vi "Display PCB coverage.vi"(0 "Inspection Data":T3, 5 "Dongle Fitted event Refnum in":T1, 11 "error in (no error)":errorcluster) -> (6 "Dongle fitted":bool, 15 "error out":errorcluster)   [LabVIEW 2013, in "Manipulate IPF.lvlib"]
uses:
  Manipulate IPF.lvlib
  type_def/but_exit.ctl
  3013/code/Modules/GUI/GUI_5/subPanels/edit/type_def/data.ctl
  3013/code/Modules/Configuration/type_def/Scan Params.ctl
  3013/code/Modules/Configuration/type_def/Profile Resolution.ctl
  3013/code/Modules/Preprocess Data/type_def/direction.ctl
  3013/code/Modules/Inspection/Data/Panel_class/type_def/Config File data.ctl
  3013/code/Modules/Inspection/type_def/Pos and Rot.ctl
  3013/code/Modules/Inspection/Data/PCB_class/type_def/PCB Params.ctl
  3013/code/Modules/Inspection/Data/Panel_class/type_def/BarCode Params.ctl
  3013/code/Modules/Barcode Reader/type_def/id.ctl
  3013/code/Modules/Inspection/Data/Panel_class/type_def/inspection data.ctl
  3013/code/Modules/Inspection/type_def/Range Limits.ctl
  Update TCF/type_def/Reload TCF_but.ctl
  type_def/Dongle fitted event refnum.ctl
  <vilib>/Utility/miscctls.llb/LVPointDoubleTypeDef.ctl
  <vilib>/Utility/cursorutil.llb/Set Cursor (Icon Pict).vi
  a3Di APG.lvlib
  3013/code/Modules/Inspection/Inspection.lvlib
  3013/code/Modules/Inspection/Data/PCB_class/PCB.lvclass
  3013/code/Modules/Barcode Reader/Barcode Reader.lvlib
  3013/code/Modules/Inspection/Data/Panel_class/Panel.lvclass
  3013/code/Modules/Configuration/Config.lvlib
  3013/code/Modules/Preprocess Data/PreProcess.lvlib
  3013/code/Modules/GUI/GUI_5/subPanels/edit/edit.lvlib
  Update TCF/TCF update.lvlib
panel:
  in  "Enable Labels":bool caption="Labels"
  out "XY Graph":cluster{dbl[], dbl[]}[](graph)
  in  "Enable Not Fited Components":bool caption="Not Fited Components"
  in  "Enable Not Tested Components":bool caption="Not Tested Components"
  in  "Save  to file":bool
  in  "Not Fitted Components":i32(listbox)
  in  "Not Tested Components":i32(listbox)
  in  "Reload":T2
  in  "Exit Button":T14
  # "Test Coverage\nComponents not tested (red), not fitted (green)"
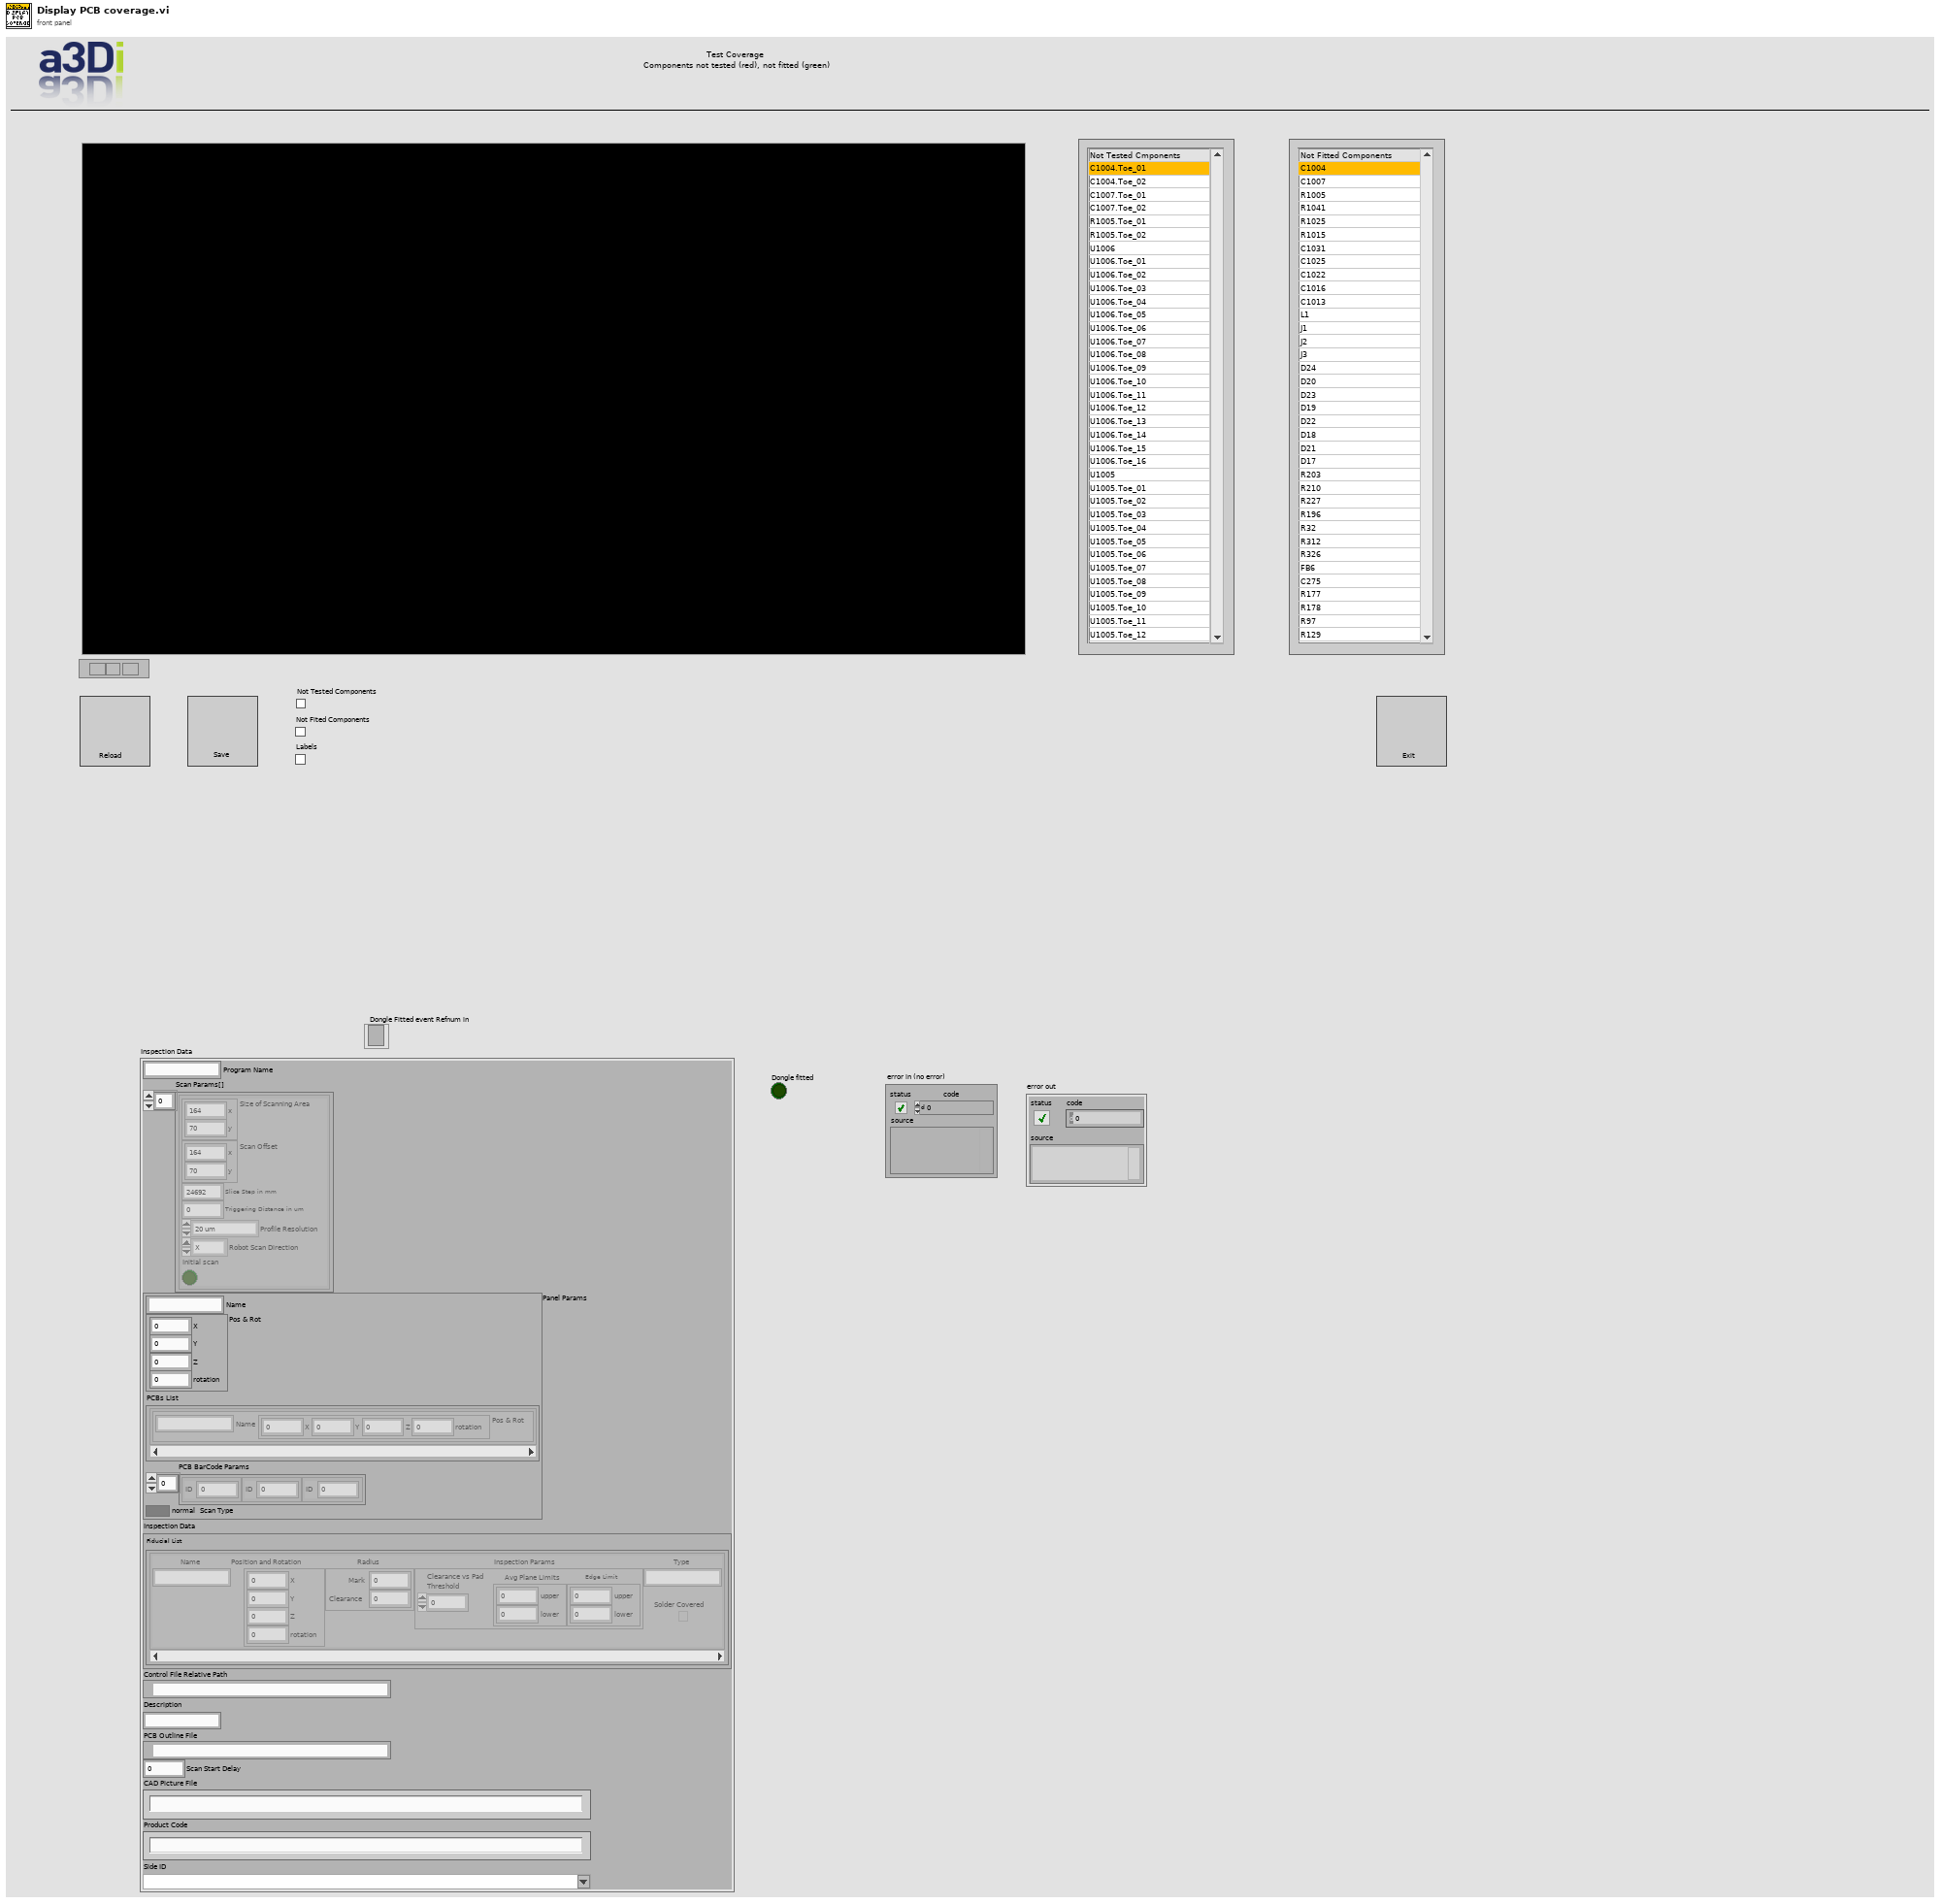
[diagram p1: front panel]
types:
  T1 = typedef "Dongle fitted event refnum.ctl" = refnum<event-registration>
  T2 = typedef "TCF update.lvlib/Reload TCF_but.ctl" = bool
  T3 = typedef "GUI.lvlib/subPanel.lvlib/edit.lvlib/data.ctl" = cluster{"Program Name":string, "Scan Params[]":T4[], "Panel Params":T7, "Inspection Data":T12, "Control File Relative Path":path, "Description":string, "PCB Outline File":path, "Scan Start Delay":dbl, "CAD Picture File":string, "Product Code":string, "Side ID":string}
  T4 = typedef "Config.lvlib/Scan Params.ctl" = cluster{"Size of Scanning Area":cluster{"x":dbl, "y":dbl}, "Scan Offset":cluster{"x":dbl, "y":dbl}, "Slice Step in mm":dbl, "Triggering Distance in mm":dbl, "Triggering Distance in um":dbl, "Profile Resolution":T5, "Version":string, "Robot Scan Direction":T6, "Initial scan":bool}
  T5 = typedef "Config.lvlib/Profile Resolution.ctl" = enum8{"20 um", "40 um"}
  T6 = typedef "PreProcess.lvlib/direction.ctl" = enum8{"X", "Y"}
  T7 = typedef "Inspection.lvlib/Panel.lvclass/Config File data.ctl" = cluster{"Name":string, "Pos & Rot":T8, "PCBs List":cluster{"PCB Params":T9}[], "PCB BarCode Params":T10[], "Scan Type":bool}
  T8 = typedef "Inspection.lvlib/Pos and Rot.ctl" = cluster{"X":dbl, "Y":dbl, "Z":dbl, "rotation":dbl}
  T9 = typedef "Inspection.lvlib/PCB.lvclass/PCB Params.ctl" = cluster{"Name":string, "Pos & Rot":T8}
  T10 = typedef "Inspection.lvlib/Panel.lvclass/BarCode Params.ctl" = cluster{"ID":T11}
  T11 = typedef "Barcode Reader.lvlib/id.ctl" = u8
  T12 = typedef "Inspection.lvlib/Panel.lvclass/inspection data.ctl" = cluster{"Fiducial List":cluster{"Name":string, "Position and Rotation":T8, "Radius":cluster{"Mark":dbl, "Clearance":dbl}, "Inspection Params":cluster{"Clearance vs Pad\nThreshold":dbl, "Avg Plane Limits":T13, "Edge Limit":T13}, "Type":string, "Solder Covered":bool}[]}
  T13 = typedef "Inspection.lvlib/Range Limits.ctl" = cluster{"upper":sgl, "lower":sgl}
  T14 = typedef "a3Di APG.lvlib/but_exit.ctl" = bool
  T15 = enum16{"Initialisation", "Wait for user input", "Scale changed", "Exit"}
  T16 = cluster{"Enable Not Tested Components":bool, "Enable Not Fited Components":bool, "Enable Labels":bool}
  T17 = enum32{"Invalid", "Standard", "Closed", "Hidden", "Minimized", "Maximized"}
  T18 = typedef "LVPointDoubleTypeDef.ctl" = cluster{"X":dbl, "Y":dbl}
  T19 = cluster{"XScale.Max":dbl, "XScale.Min":dbl, "YScale.Max":dbl, "YScale.Min":dbl}
  T20 = cluster{"Not fitted components":string[], "Not tested components":string[], "Not Fitted position[x][y] ":dbl[][], "Not Tested position[x][y]":dbl[][], "CAD Layers":cluster{"1st Filtered Array out":sgl[], "2nd Filtered Array out":sgl[]}[], "Xyz File Exist? ":bool, "Options":cluster{"Enable Not Tested Components":bool, "Enable Not Fited Components":bool, "Enable Labels":bool}, "Origin XY Scale Ranges":cluster{"XScale.Max":dbl, "XScale.Min":dbl, "YScale.Max":dbl, "YScale.Min":dbl}}
  T21 = typedef "LVPoint32TypeDef.ctl" = cluster{"Horizontal":i32, "Vertical":i32}
  T22 = cluster{"XScale.Offset":dbl, "YScale.Offset":dbl}
  T23 = cluster{"XScale.Multiplier":dbl, "YScale.Multiplier":dbl}
  T24 = typedef "LVAnnotationListTypeDef.ctl" = cluster{"Name":string, "Color":u32, "Style":u8, "Point Style":u8, "Name Visible":bool, "Allow Drag":bool, "Annotation Mode":u32, "Plot":i32, "Index":i32, "Position":cluster{"X":dbl, "Y":dbl}, "X Scale":u32, "Y Scale":u32, "Show Arrow":bool, "Lock Name":bool, "Plot Area":i32, "Label Offset":cluster{"X":dbl, "Y":dbl}}[]
  T25 = cluster{"Name":string, "Color":u32, "Style":u8, "Point Style":u8, "Name Visible":bool, "Allow Drag":bool, "Annotation Mode":u32, "Plot":i32, "Index":i32, "Position":cluster{"X":dbl, "Y":dbl}, "X Scale":u32, "Y Scale":u32, "Show Arrow":bool, "Lock Name":bool, "Plot Area":i32, "Label Offset":cluster{"X":dbl, "Y":dbl}}
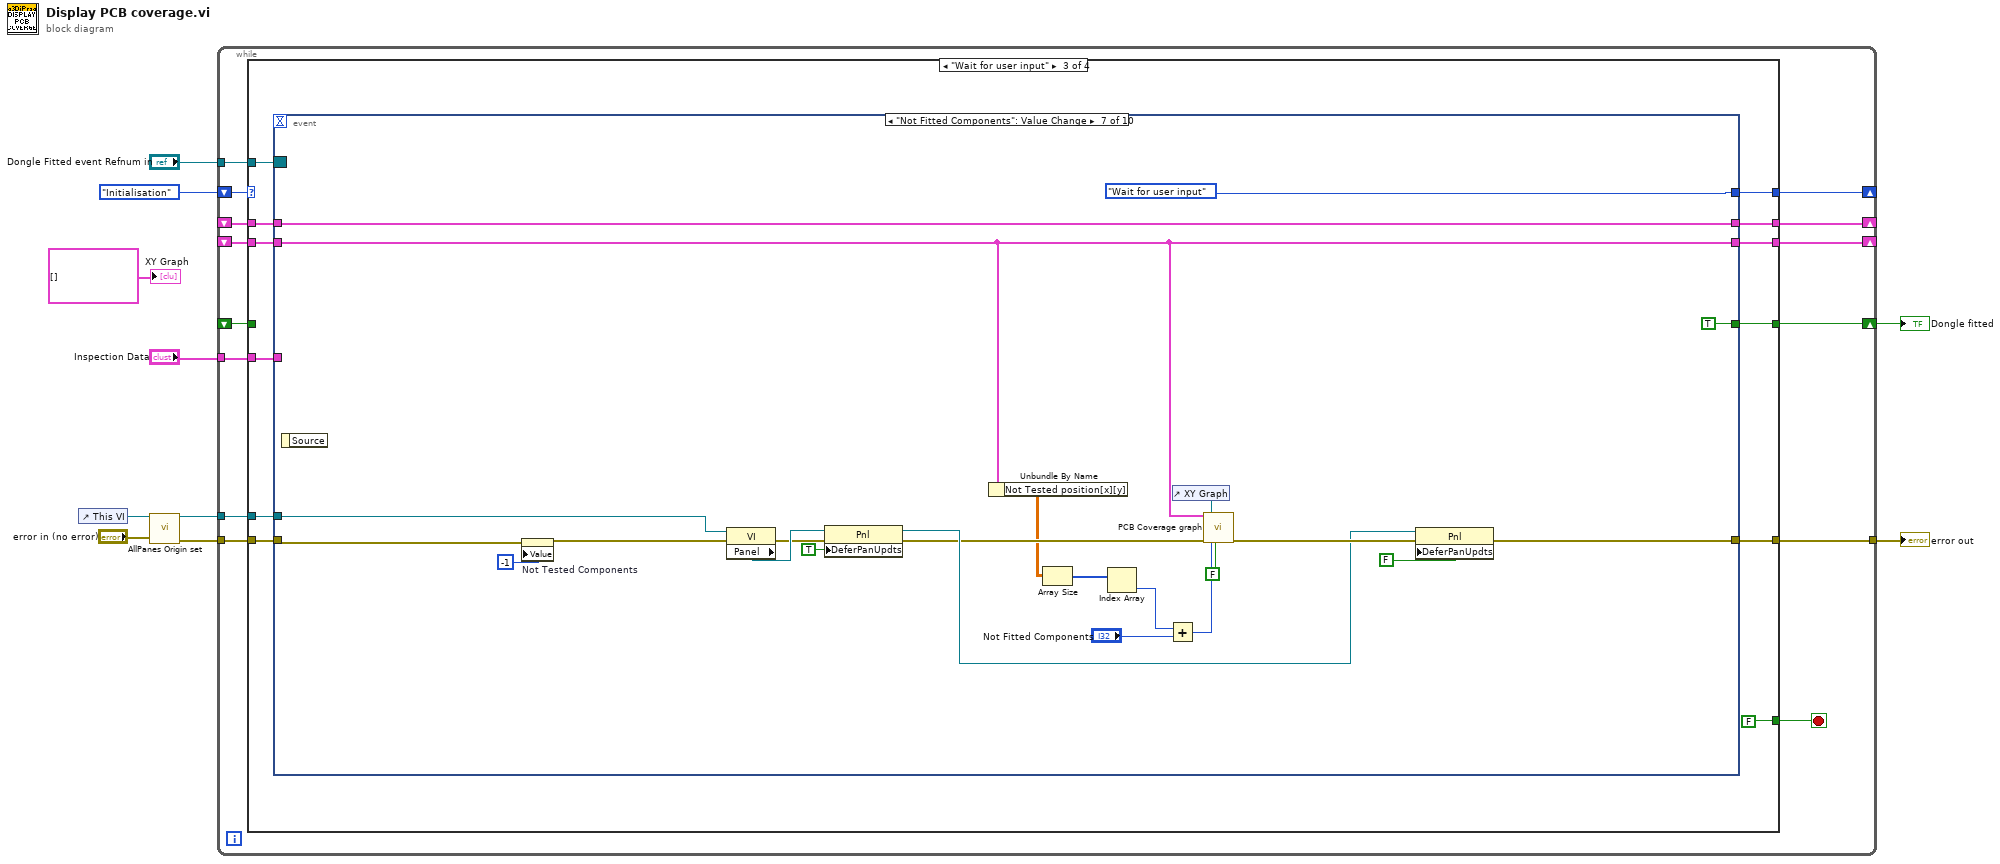
[diagram p0: block diagram]
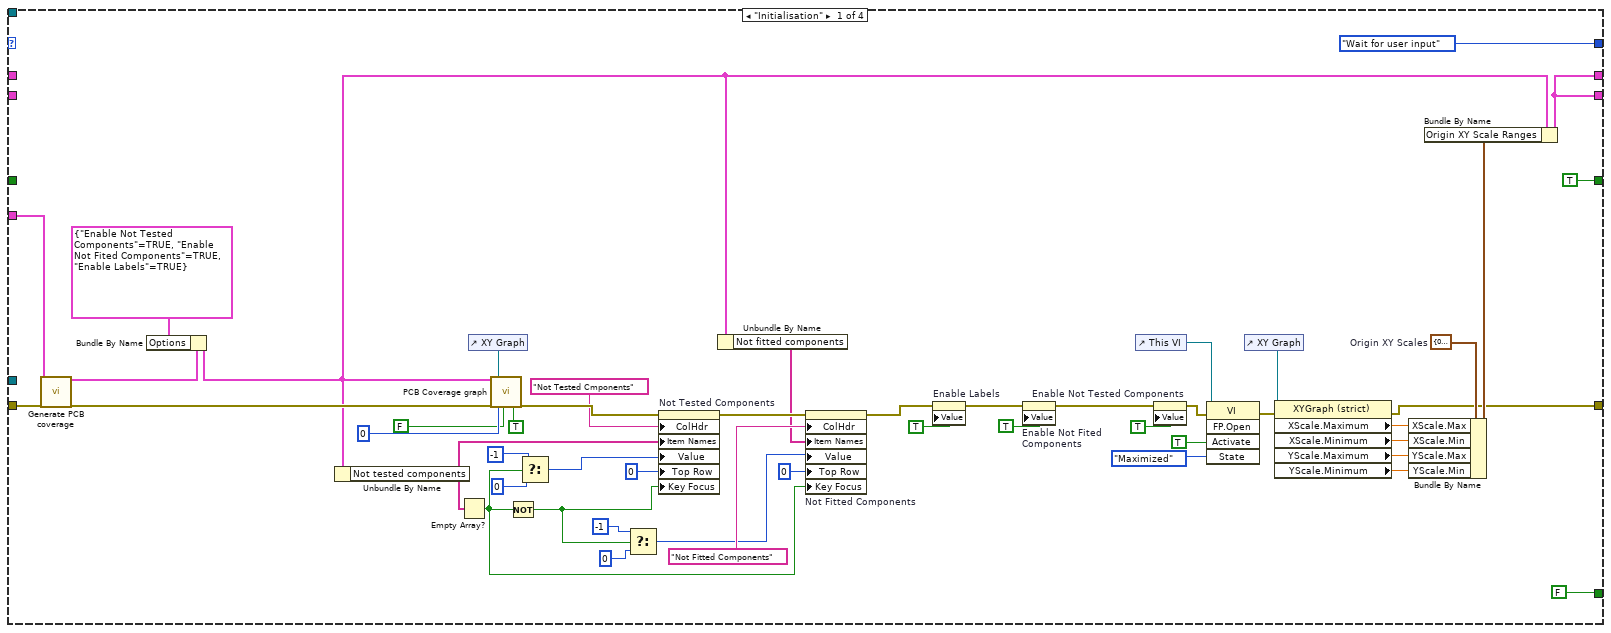
[diagram p2: hidden frame]
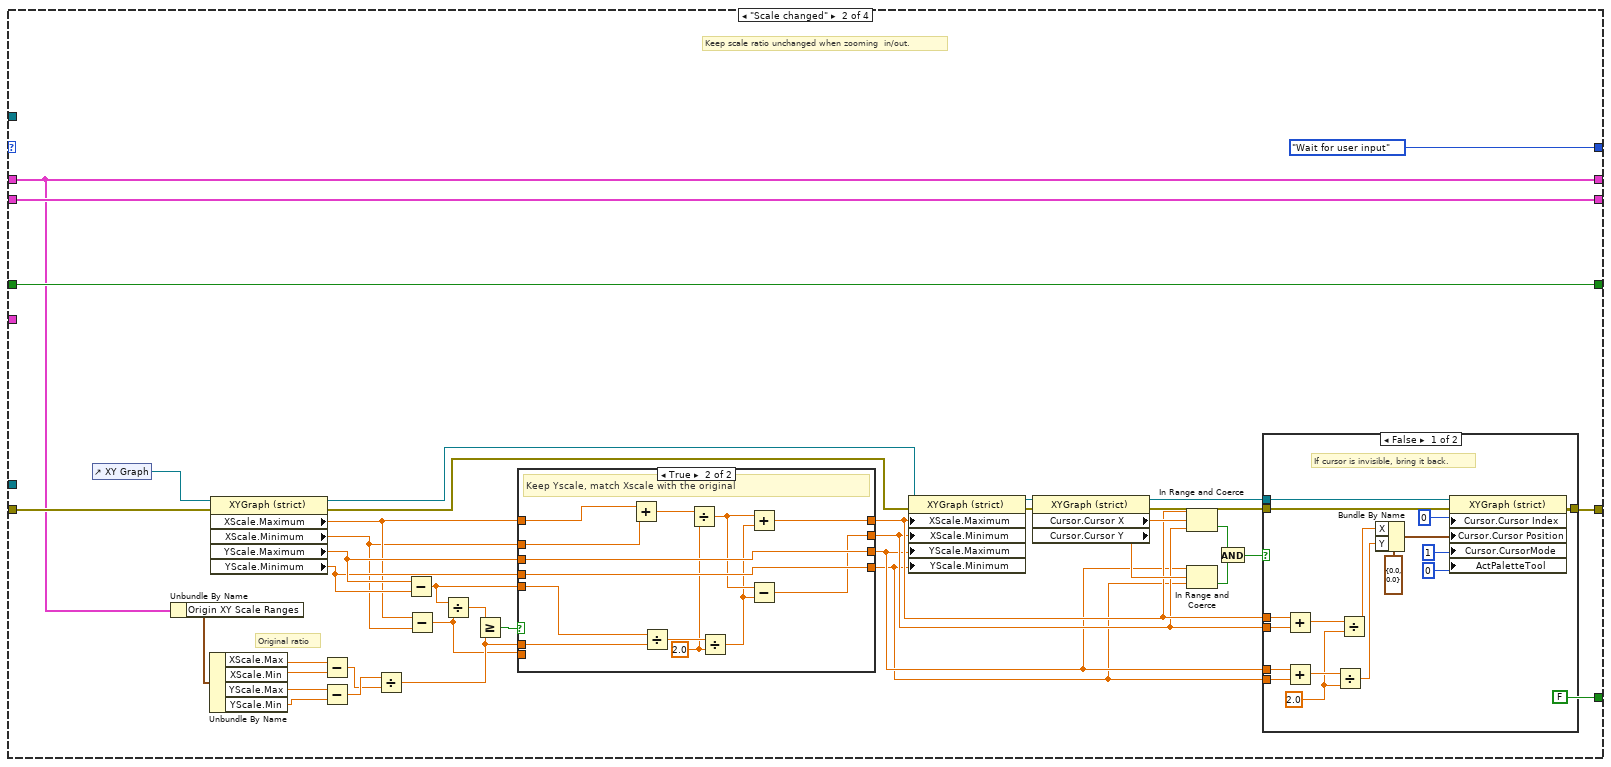
[diagram p3: hidden frame]
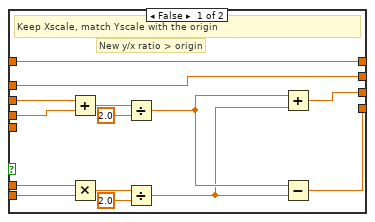
[diagram p5: hidden frame]
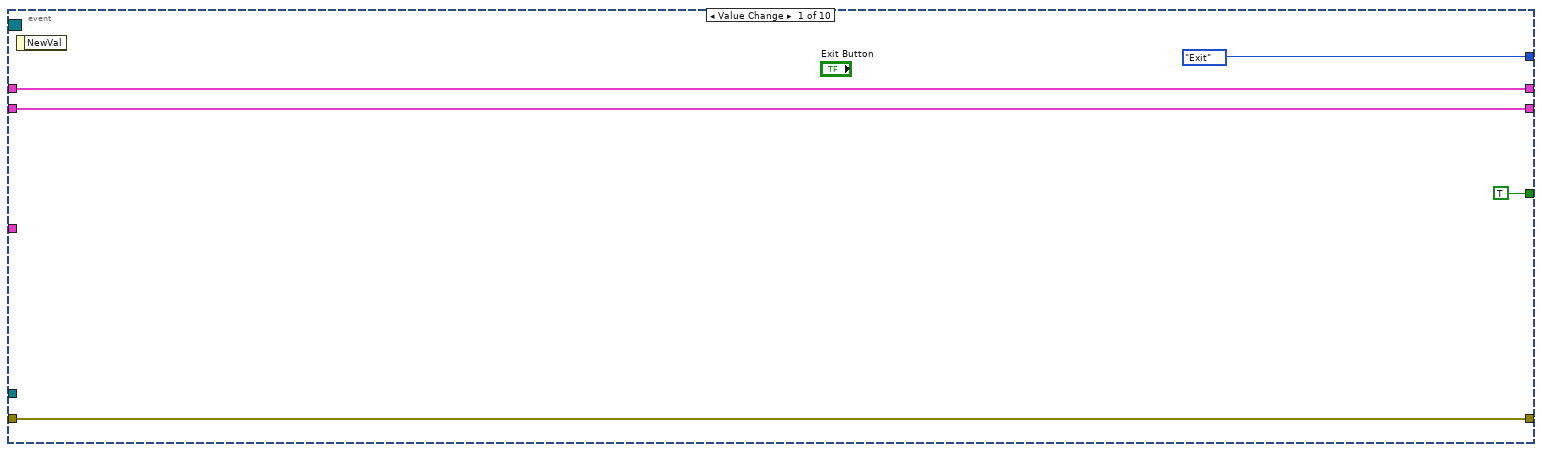
[diagram p6: hidden frame]
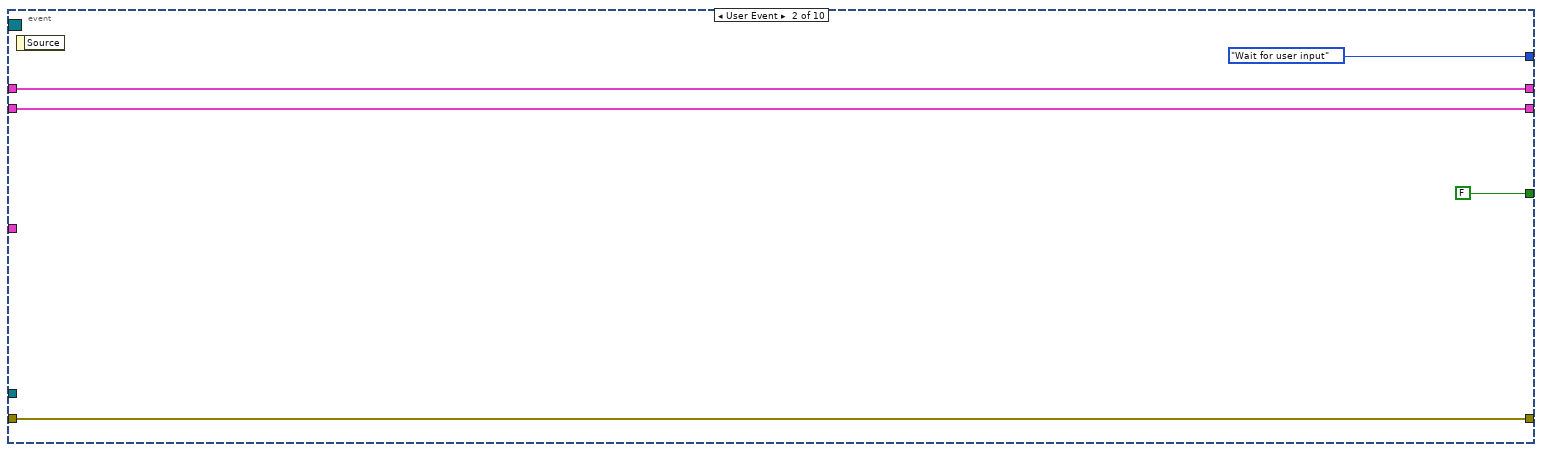
[diagram p7: hidden frame]
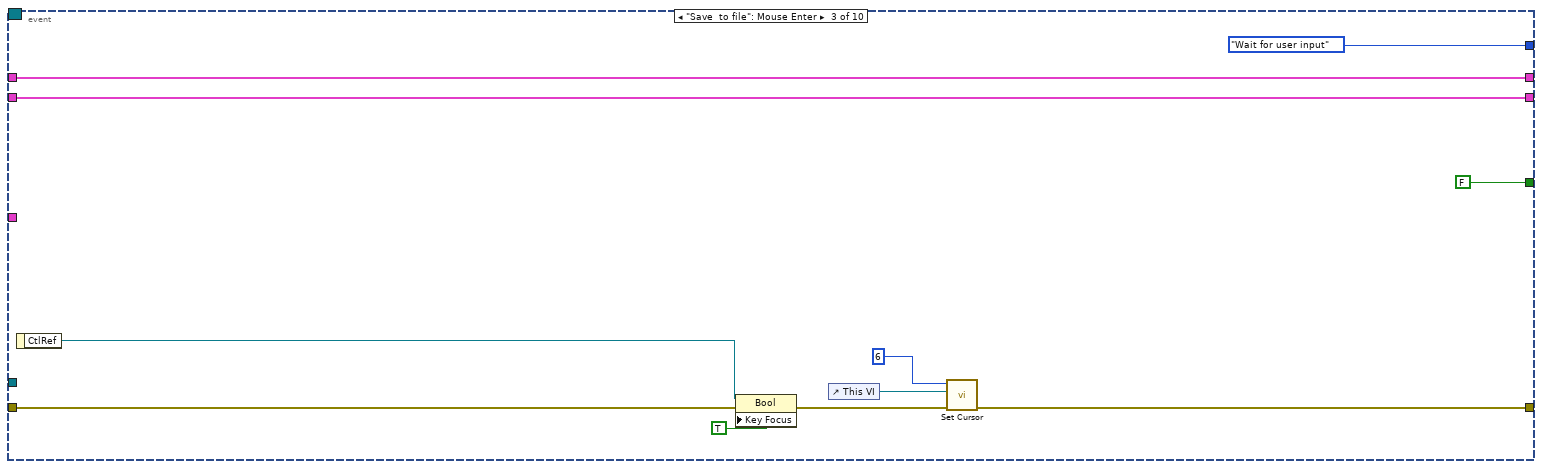
[diagram p8: hidden frame]
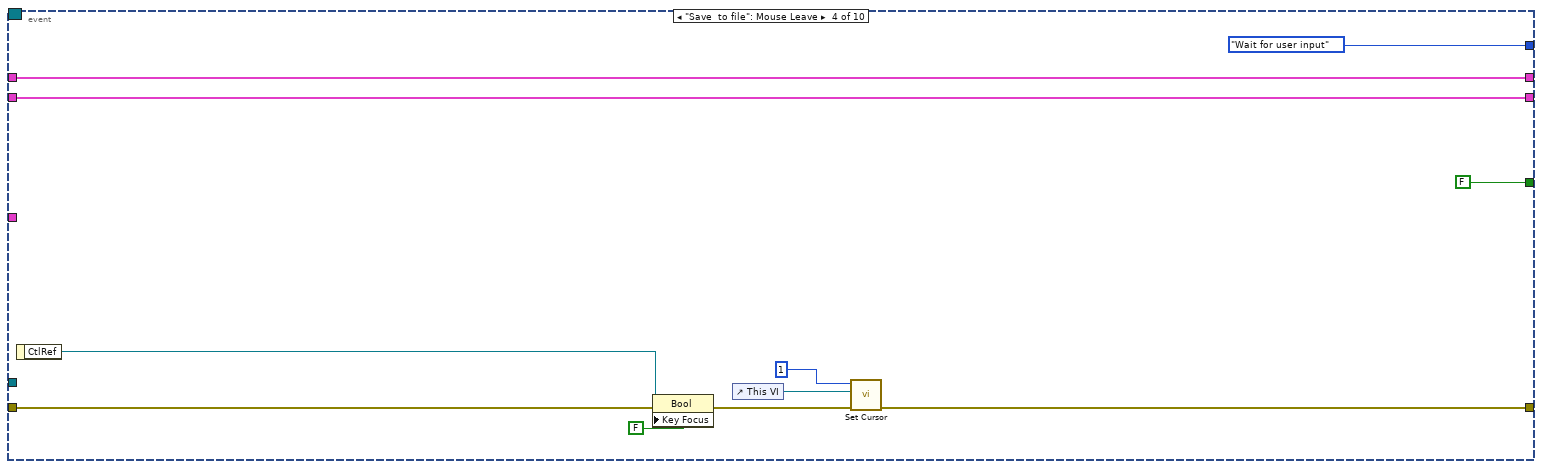
[diagram p9: hidden frame]
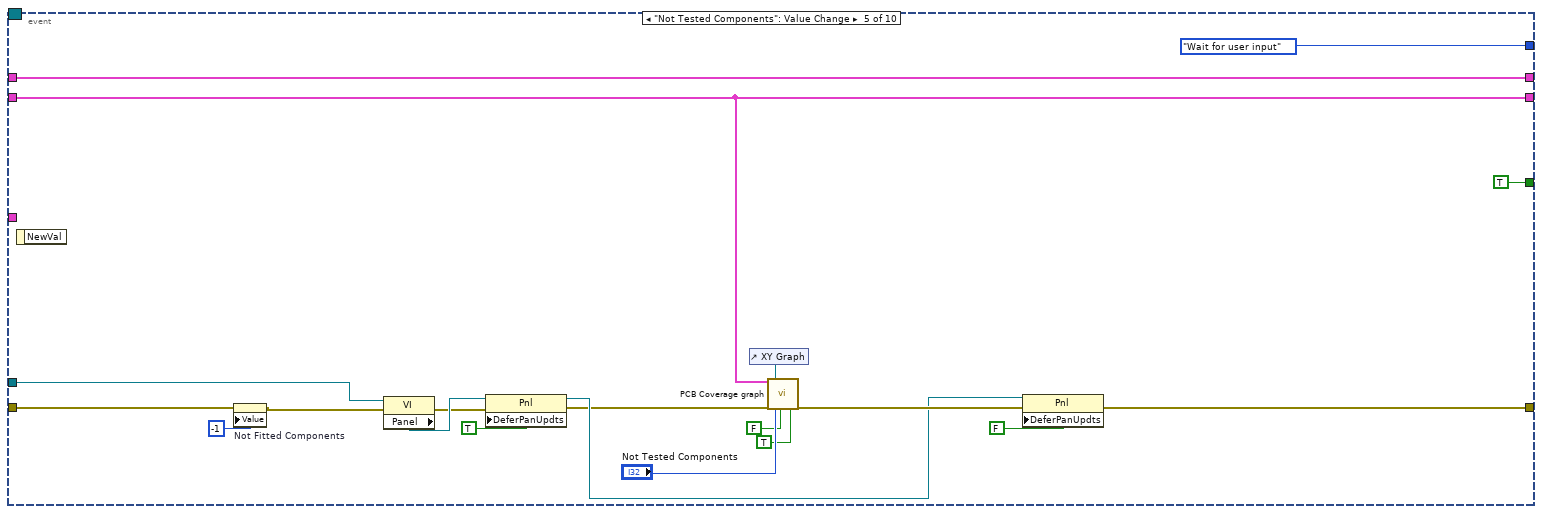
[diagram p10: hidden frame]
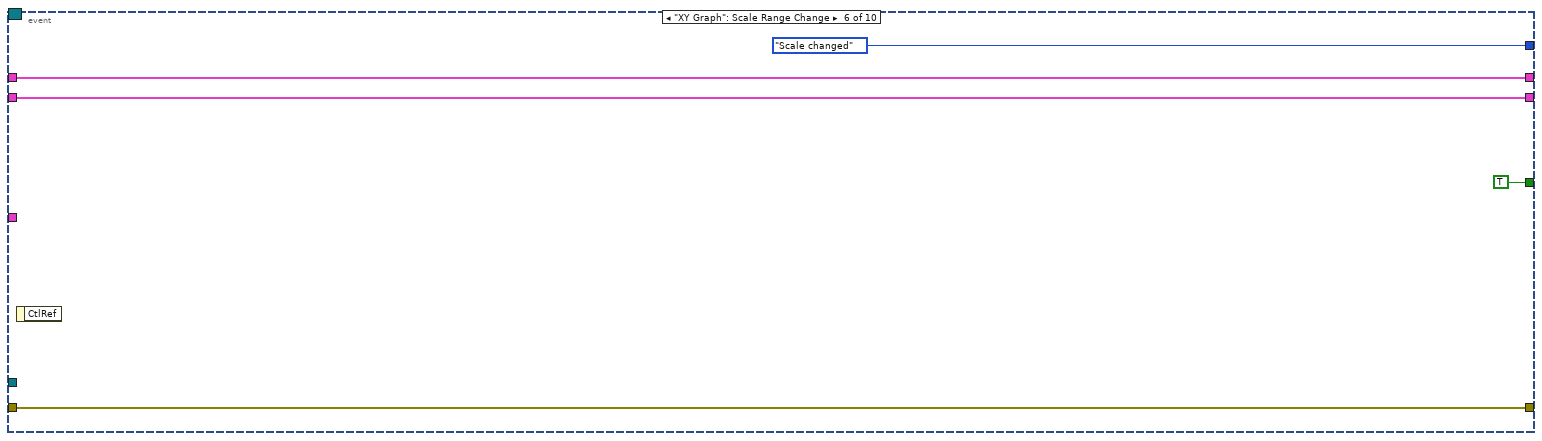
[diagram p11: hidden frame]
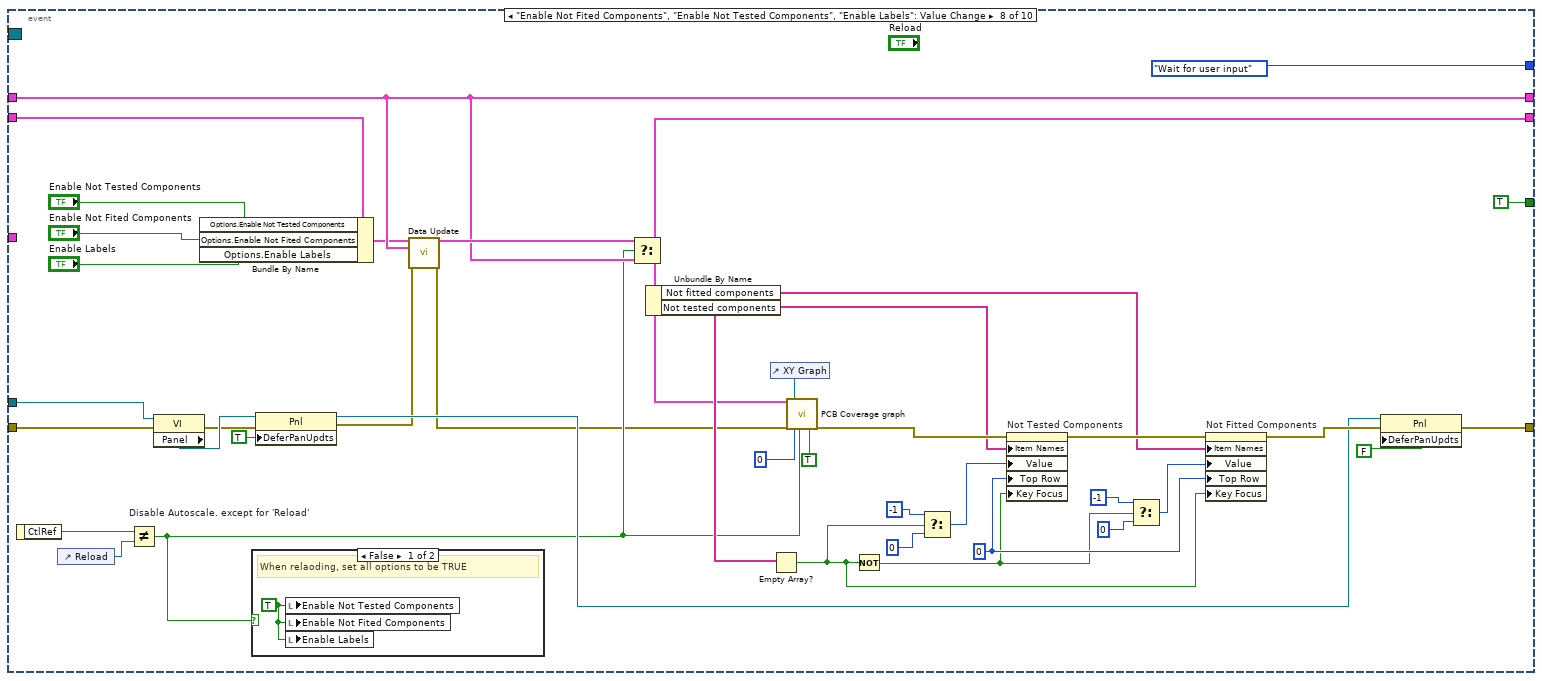
[diagram p12: hidden frame]
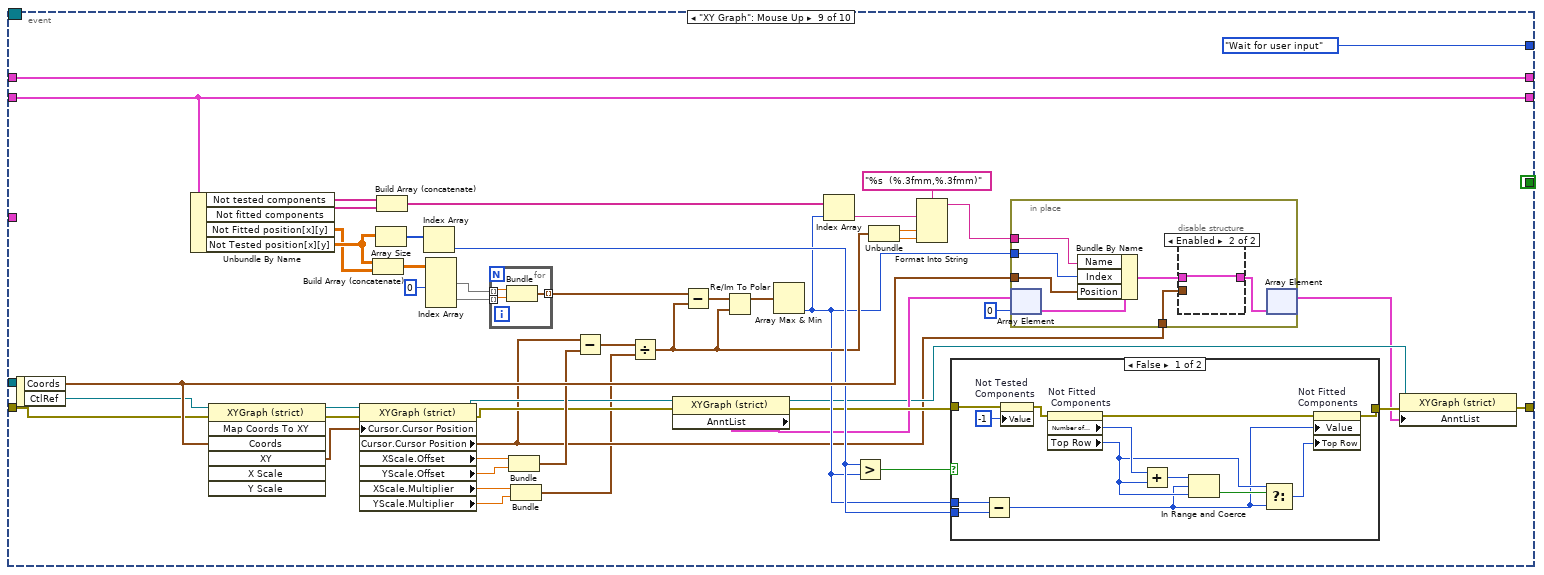
[diagram p14: hidden frame]
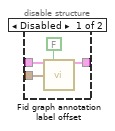
[diagram p15: hidden frame]
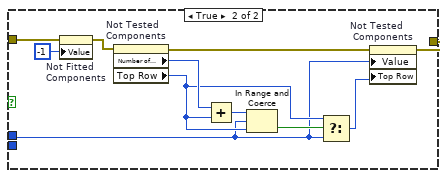
[diagram p16: hidden frame]
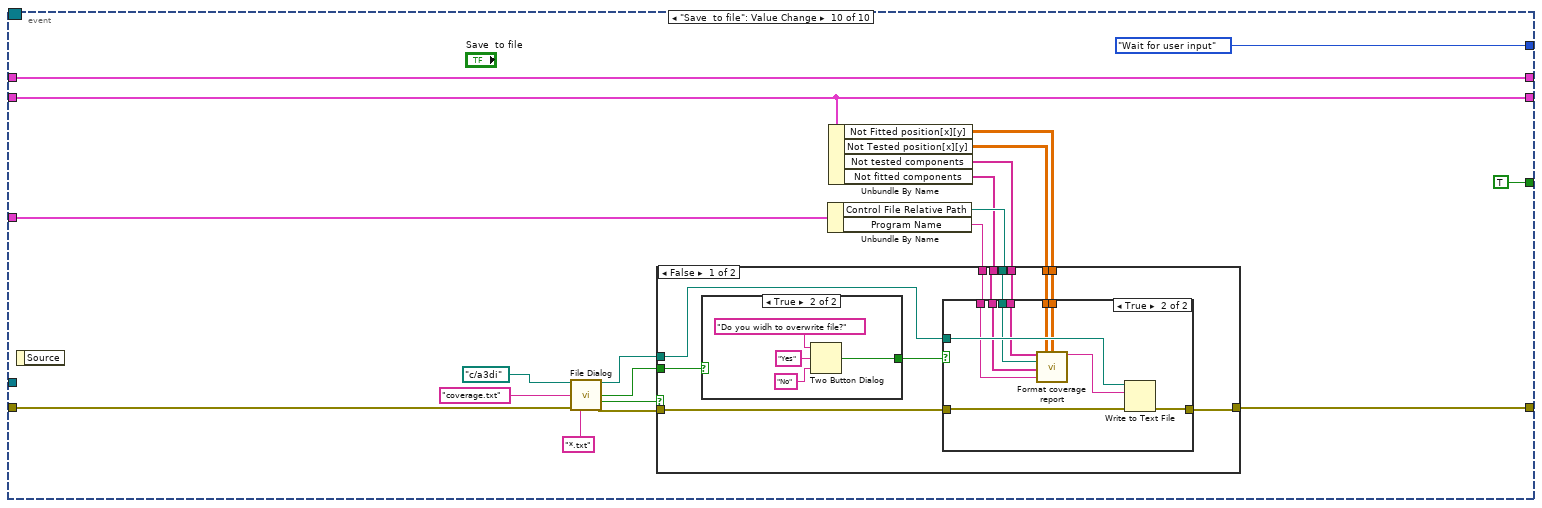
[diagram p17: hidden frame]
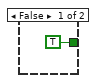
[diagram p19: hidden frame]
diagram:
  n1 = control-ref of="This VI"() -> (w10:refnum<vi>)
  n2 = call "AllPanes Origin set.vi"("VI ref in"=w10, "error in"="error in (no error)") -> ("VI ref out"=w7:refnum<vi>, "error out"=w8:errorcluster)  [unwired: 12 in]
  n3 = while {
    tunnel: w8 -> [w22]
    shift-right: [w23] -> _
    shift-left: T15."Initialisation" -> [w24]
    tunnel: [w19] -> w1
    tunnel: w7 -> [w21]
    tunnel: "Inspection Data" -> [w20]
    tunnel: "Dongle Fitted event Refnum in" -> [w18]
    shift-right: [w17] -> w4
    shift-left: _ -> [w16]
    shift-right: [w15] -> _
    shift-left: _ -> [w14]
    shift-right: [w12] -> _
    shift-left: _ -> [w13]
    stop <- w11 stop-if-true
    n4 = case shown="\"Wait for user input\"" w24 {
      tunnel: [FALSE FALSE FALSE TRUE] -> w11
      tunnel: [T15."Wait for user input" T15."Wait for user input" w169 T15."Exit"] -> w23
      tunnel: w22 -> [w34 w109 w167 w433]
      tunnel: [w25 w87 w158 w427] -> w19
      tunnel: w21 -> [_ _ w163 w432]
      tunnel: w20 -> [w69 _ w168 _]
      tunnel: w18 -> [_ _ w165 _]
      tunnel: [TRUE w111 w164 w431] -> w17
      tunnel: w16 -> [_ w111 _ w431]
      tunnel: [w27 w107 w161 w429] -> w15
      tunnel: w14 -> [_ w107 w162 w429]
      tunnel: w13 -> [_ w108 w159 w428]
      tunnel: [w27 w108 w160 w428] -> w12
      frame "Initialisation" {
        w41 = T19 {"XScale.Max"=0.0, "XScale.Min"=0.0, "YScale.Max"=0.0, "YScale.Min"=0.0}  # Origin XY Scales
        n5 = call "Generate PCB coverage.vi"("Inspection Data"=w69, "error in (no error)"=w34) -> ("DataOut"=w31:T20, "error out"=w68:errorcluster)  [unwired: 16 in]
        n6 = Bundle By Name(cluster=w31, "Options"=T16 {"Enable Not Tested Components"=TRUE, "Enable Not Fited Components"=TRUE, "Enable Labels"=TRUE}) -> (w29:T20)
        n7 = Unbundle By Name(w29) -> ("Not tested components"=w28:string[])
        n8 = Empty Array?(array=w28) -> (empty?=w54:bool)
        n9 = control-ref of="XY Graph"() -> (w47:refnum<vi>)
        n10 = call "PCB Coverage graph.vi"("UpdatedData"=w29, "error in (no error)"=w68, "XY Graph"=w47, "index"=0, "Disable Autoscale"=FALSE ("Disable Zoom Back?"), "Initialise graph"=TRUE) -> ("error out"=w67:errorcluster)  [unwired: 13 in]
        n11 = Not(x=w54) -> (.not. x?=w57:bool)
        n12 = Select(t=-1 ("Not Tested Components"), s=w54, f=0 ("Not Tested Components")) -> (s? t:f=w59:i32)
        n13 = Select(t=-1 ("Not Tested Components"), s=w57, f=0 ("Not Tested Components")) -> (s? t:f=w55:i32)
        n14 = property on="Not Tested Components" class="LstBox (strict)"(error in=w67, "ColHdr"="Not Tested Cmponents" ("Column Header String"), "Item Names"=w28, "Value"=w59, "Top Row"=0 ("Not Tested Components"), "Key Focus"=w57) -> (error out=w66:errorcluster)  [unwired: 1 in, 1 out]
        n15 = Unbundle By Name(w29) -> ("Not fitted components"=w30:string[])
        n16 = property on="Not Fitted Components" class="LstBox (strict)"(error in=w66, "ColHdr"="Not Fitted Components" ("Column Header String"), "Item Names"=w30, "Value"=w55, "Top Row"=0 ("Not Fitted Components"), "Key Focus"=w54) -> (error out=w46:errorcluster)  [unwired: 1 in, 1 out]
        n17 = property on="Enable Labels" class="Bool (strict)"(error in=w46, "Value"=TRUE ("Enable Labels")) -> (error out=w45:errorcluster)  [unwired: 1 in, 1 out]
        n18 = property on="Enable Not Fited Components" class="Bool (strict)"(error in=w45, "Value"=TRUE ("Not Fited Components")) -> (error out=w49:errorcluster)  [unwired: 1 in, 1 out]
        n19 = control-ref of="This VI"() -> (w70:refnum<vi>)
        n20 = property on="Enable Not Tested Components" class="Bool (strict)"(error in=w49, "Value"=TRUE ("Not Fited Components")) -> (error out=w48:errorcluster)  [unwired: 1 in, 1 out]
        n21 = invoke class="VI" method="FP.Open"(reference=w70, error in=w48, "Activate"=TRUE ("Activate?"), "State"=T17."Maximized") -> (error out=w35:errorcluster)  [unwired: 1 in, 4 out]
        n22 = control-ref of="XY Graph"() -> (w42:refnum<vi>)
        n23 = property class="XYGraph (strict)"(reference=w42, error in=w35) -> (error out=w25:errorcluster, "XScale.Maximum"=w40:dbl, "XScale.Minimum"=w39:dbl, "YScale.Maximum"=w38:dbl, "YScale.Minimum"=w37:dbl)  [unwired: 1 out]
        n24 = Bundle By Name(cluster=w41, "XScale.Max"=w40, "XScale.Min"=w39, "YScale.Max"=w38, "YScale.Min"=w37) -> (w26:T19)
        n25 = Bundle By Name(cluster=w29, "Origin XY Scale Ranges"=w26) -> (w27:T20)
      }
      frame "Scale changed" {
        # "Original ratio"
        # "Keep scale ratio unchanged when zooming  in/out."
        n26 = control-ref of="XY Graph"() -> (w106:refnum<vi>)
        n27 = Unbundle By Name(w107) -> ("Origin XY Scale Ranges"=w88:T19)
        n28 = Unbundle By Name(w88) -> ("XScale.Max"=w104:dbl, "XScale.Min"=w103:dbl, "YScale.Max"=w102:dbl, "YScale.Min"=w101:dbl)
        n29 = property class="XYGraph (strict)"(reference=w106, error in=w109) -> (reference out=w105:refnum<vi>, error out=w89:errorcluster, "XScale.Maximum"=w94:dbl, "XScale.Minimum"=w93:dbl, "YScale.Maximum"=w96:dbl, "YScale.Minimum"=w95:dbl)
        n30 = Subtract(x=w104, y=w103) -> (x-y=w99:dbl)
        n31 = Subtract(x=w102, y=w101) -> (x-y=w100:dbl)
        n32 = Divide(x=w100, y=w99) -> (x/y=w92:dbl)
        n33 = Subtract(x=w96, y=w95) -> (x-y=w91:dbl)
        n34 = Subtract(x=w94, y=w93) -> (x-y=w90:dbl)
        n35 = Divide(x=w91, y=w90) -> (x/y=w98:dbl)
        n36 = Greater Or Equal?(x=w98, y=w92) -> (x >= y?=w97:bool)
        n37 = case shown="True" w97 {
          tunnel: w96 -> [w137 w157]
          tunnel: [w142 w157] -> w78
          tunnel: [w131 w156] -> w77
          tunnel: w95 -> [w136 w156]
          tunnel: w94 -> [w144 w152]
          tunnel: [w144 w149] -> w80
          tunnel: w93 -> [w143 w151]
          tunnel: [w143 w146] -> w79
          tunnel: w92 -> [w140 w154]
          tunnel: w91 -> [_ w155]
          tunnel: w90 -> [w141 _]
          frame False {
            # "New y/x ratio > origin"
            # "Keep Xscale, match Yscale with the origin"
            n38 = Add(x=w137, y=w136) -> (x+y=w134:dbl)
            n39 = Multiply(x=w140, y=w141) -> (x*y=w139:dbl)
            n40 = Divide(x=w134, y=2.0) -> (x/y=w133:dbl)
            n41 = Divide(x=w139, y=2.0) -> (x/y=w132:dbl)
            n42 = Add(x=w133, y=w132) -> (x+y=w142:dbl)
            n43 = Subtract(x=w133, y=w132) -> (x-y=w131:dbl)
          }
          frame True {
            w145 = 2.0 ("y")
            # "Keep Yscale, match Xscale with the original"
            n44 = Add(x=w152, y=w151) -> (x+y=w150:dbl)
            n45 = Divide(x=w155, y=w154) -> (x/y=w153:dbl)
            n46 = Divide(x=w150, y=w145) -> (x/y=w148:dbl)
            n47 = Divide(x=w153, y=w145) -> (x/y=w147:dbl)
            n48 = Add(x=w148, y=w147) -> (x+y=w149:dbl)
            n49 = Subtract(x=w148, y=w147) -> (x-y=w146:dbl)
          }
        }
        n50 = property class="XYGraph (strict)"(reference=w105, error in=w89, "XScale.Maximum"=w80, "XScale.Minimum"=w79, "YScale.Maximum"=w78, "YScale.Minimum"=w77) -> (reference out=w86:refnum<vi>, error out=w84:errorcluster)
        n51 = property class="XYGraph (strict)"(reference=w86, error in=w84) -> (reference out=w85:refnum<vi>, error out=w83:errorcluster, "Cursor.Cursor X"=w82:dbl, "Cursor.Cursor Y"=w81:dbl)
        n52 = In Range and Coerce(upper limit=w80, x=w82, lower limit=w79) -> (In Range?=w76:bool)  [unwired: 1 out]
        n53 = In Range and Coerce(upper limit=w78, x=w81, lower limit=w77) -> (In Range?=w75:bool)  [unwired: 1 out]
        n54 = And(x=w76, y=w75) -> (x .and. y?=w74:bool)
        n55 = case shown="False" w74 {
          tunnel: w80 -> [w124 _]
          tunnel: w79 -> [w123 _]
          tunnel: w78 -> [w119 _]
          tunnel: w77 -> [w118 _]
          tunnel: [w116 w130] -> w87
          tunnel: w85 -> [w114 _]
          tunnel: w83 -> [w113 w130]
          frame False {
            w115 = 2.0 ("y")
            # "If cursor is invisible, bring it back."
            n56 = Add(x=w124, y=w123) -> (x+y=w122:dbl)
            n57 = Add(x=w119, y=w118) -> (x+y=w120:dbl)
            n58 = Divide(x=w120, y=w115) -> (x/y=w117:dbl)
            n59 = Divide(x=w122, y=w115) -> (x/y=w121:dbl)
            n60 = Bundle By Name(cluster=T18 {"X"=0.0, "Y"=0.0} ("Cursor.Cursor Position"), "X"=w121, "Y"=w117) -> (w126:T18)
            n61 = property class="XYGraph (strict)"(reference=w114, error in=w113, "Cursor.Cursor Index"=0, "Cursor.Cursor Position"=w126, "Cursor.CursorMode"=u32 1 ("Cursor.Cursor Mode"), "ActPaletteTool"=0 ("Palette:Active Tool")) -> (error out=w116:errorcluster)  [unwired: 1 out]
          }
          frame True {
          }
        }
      }
      frame "Wait for user input" {
        n62 = event shown="[6] \"Not Fitted Components\": Value Change" {
          selector: w165 -> [_ _ _ _ _ _ _ _ _ _]
          dyn-events: _ -> [_ _ _ _ _ _ _ _ _ _]
          timeout: _ -> [_ _ _ _ _ _ _ _ _ _]
          tunnel: [T15."Exit" T15."Wait for user input" T15."Wait for user input" T15."Wait for user input" T15."Wait for user input" T15."Scale changed" T15."Wait for user input" T15."Wait for user input" T15."Wait for user input" T15."Wait for user input"] -> w169
          tunnel: w168 -> [_ _ _ _ _ _ _ _ _ w389]
          tunnel: w167 -> [w174 w179 w181 w192 w210 w222 w235 w252 w291 w398]
          tunnel: [w174 w179 w185 w196 w214 w222 w239 w284 w292 w393] -> w158
          tunnel: w163 -> [_ _ _ _ w216 _ w241 w289 _ _]
          tunnel: [TRUE FALSE FALSE FALSE TRUE TRUE TRUE TRUE TRUE TRUE] -> w164
          tunnel: w162 -> [w171 w176 w188 w199 w202 w224 w229 w260 w336 w384]
          tunnel: [w171 w176 w188 w199 w202 w224 w229 w260 w336 w384] -> w161
          tunnel: [w170 w175 w187 w198 w203 w223 w228 w261 w293 w383] -> w160
          tunnel: w159 -> [w170 w175 w187 w198 w203 w223 w228 w257 w293 w383]
          event Value Change {
            n63 = event-data() -> ()  [unwired: 1 in, 1 out]
          }
          event User Event {
            n64 = event-data() -> ()  [unwired: 1 in, 1 out]
          }
          event "Save  to file": Mouse Enter {
            n65 = event-data() -> ("CtlRef"=w183:refnum<vi>)  [unwired: 1 in]
            n66 = property class="Bool"(reference=w183, error in=w181, "Key Focus"=TRUE) -> (error out=w180:errorcluster)  [unwired: 1 out]
            n67 = control-ref of="This VI"() -> (w186:refnum<vi>)
            n68 = call-poly <vilib>:"Set Cursor.vi"("error in (no error)"=w180, "VI reference (current VI)"=w186, "icon"=u16 6) -> ("error out"=w185:errorcluster)  [unwired: 7 in, 1 out]
          }
          event "Save  to file": Mouse Leave {
            n69 = event-data() -> ("CtlRef"=w194:refnum<vi>)  [unwired: 1 in]
            n70 = property class="Bool"(reference=w194, error in=w192, "Key Focus"=FALSE) -> (error out=w191:errorcluster)  [unwired: 1 out]
            n71 = control-ref of="This VI"() -> (w197:refnum<vi>)
            n72 = call-poly <vilib>:"Set Cursor.vi"("error in (no error)"=w191, "VI reference (current VI)"=w197, "icon"=u16 1) -> ("error out"=w196:errorcluster)  [unwired: 7 in, 1 out]
          }
          event "Not Tested Components": Value Change {
            n73 = event-data() -> ()  [unwired: 1 in, 1 out]
            n74 = property on="Not Fitted Components" class="LstBox (strict)"(error in=w210, "Value"=-1 ("Not Fitted Components")) -> (error out=w209:errorcluster)  [unwired: 1 in, 1 out]
            n75 = property class="VI"(reference=w216, error in=w209) -> (error out=w218:errorcluster, "Panel"=w219:refnum<vi>)  [unwired: 1 out]
            n76 = property class="Pnl"(reference=w219, error in=w218, "DeferPanUpdts"=TRUE ("Defer Panel Updates")) -> (reference out=w212:refnum<vi>, error out=w211:errorcluster)
            n77 = control-ref of="XY Graph"() -> (w207:refnum<vi>)
            n78 = call "PCB Coverage graph.vi"("UpdatedData"=w203, "error in (no error)"=w211, "XY Graph"=w207, "index"="Not Tested Components", "Disable Autoscale"=FALSE ("Disable Zoom Back?"), "Initialise graph"=TRUE) -> ("error out"=w215:errorcluster)  [unwired: 13 in]
            n79 = property class="Pnl"(reference=w212, error in=w215, "DeferPanUpdts"=FALSE ("Defer Panel Updates")) -> (error out=w214:errorcluster)  [unwired: 1 out]
          }
          event "XY Graph": Scale Range Change {
            n80 = event-data() -> ()  [unwired: 1 in, 1 out]
          }
          event "Not Fitted Components": Value Change {
            n81 = event-data() -> ()  [unwired: 1 in, 1 out]
            n82 = property on="Not Tested Components" class="LstBox (strict)"(error in=w235, "Value"=-1 ("Not Fitted Components")) -> (error out=w234:errorcluster)  [unwired: 1 in, 1 out]
            n83 = property class="VI"(reference=w241, error in=w234) -> (error out=w243:errorcluster, "Panel"=w244:refnum<vi>)  [unwired: 1 out]
            n84 = property class="Pnl"(reference=w244, error in=w243, "DeferPanUpdts"=TRUE ("Defer Panel Updates")) -> (reference out=w237:refnum<vi>, error out=w236:errorcluster)
            n85 = Unbundle By Name(w228) -> ("Not Tested position[x][y]"=w227:dbl[][])
            n86 = Array Size(array=w227) -> (size(s)=w248:i32[])
            n87 = Index Array(array=w248) -> (element=w247:i32)  [unwired: 1 in]
            n88 = Add(x=w247, y="Not Fitted Components") -> (x+y=w245:i32)
            n89 = control-ref of="XY Graph"() -> (w232:refnum<vi>)
            n90 = call "PCB Coverage graph.vi"("UpdatedData"=w228, "error in (no error)"=w236, "XY Graph"=w232, "index"=w245, "Disable Autoscale"=FALSE ("Disable Zoom Back?")) -> ("error out"=w240:errorcluster)  [unwired: 14 in]
            n91 = property class="Pnl"(reference=w237, error in=w240, "DeferPanUpdts"=FALSE ("Defer Panel Updates")) -> (error out=w239:errorcluster)  [unwired: 1 out]
          }
          event "Enable Not Fited Components", "Enable Not Tested Components", "Enable Labels": Value Change {
            w279 = 0 ("index")
            n92 = event-data() -> ("CtlRef"=w267:refnum<vi>)  [unwired: 1 in]
            n93 = control-ref of="Reload"() -> (w265:refnum<vi>)
            n94 = Not Equal? "Disable Autoscale. except for 'Reload'"(x=w267, y=w265) -> (x != y?=w258:bool)
            n95 = property class="VI"(reference=w289, error in=w252) -> (error out=w287:errorcluster, "Panel"=w288:refnum<vi>)  [unwired: 1 out]
            n96 = Bundle By Name(cluster=w257, "Options.Enable Not Tested Components"="Enable Not Tested Components", "Options.Enable Not Fited Components"="Enable Not Fited Components", "Options.Enable Labels"="Enable Labels") -> (w256:T20)
            n97 = case shown="False" w258 {
              frame False {
                w290 = TRUE ("Enable Not Tested Components")
                # "When relaoding, set all options to be TRUE"
                n98 = local write "Enable Not Tested Components"(w290) -> ()
                n99 = local write "Enable Not Fited Components"(w290) -> ()
                n100 = local write "Enable Labels"(w290) -> ()
              }
              frame True {
              }
            }
            n101 = property class="Pnl"(reference=w288, error in=w287, "DeferPanUpdts"=TRUE ("Defer Panel Updates")) -> (reference out=w282:refnum<vi>, error out=w251:errorcluster)
            n102 = call "Data Update.vi"("UpdatedDataIn"=w256, "OriginData"=w260, "error in (no error)"=w251) -> ("UpdateDataOut"=w262:T20, "error out"=w250:errorcluster)  [unwired: 11 in]
            n103 = Select(t=w262, s=w258, f=w260) -> (s? t:f=w261:T20)
            n104 = Unbundle By Name(w261) -> ("Not fitted components"=w259:string[], "Not tested components"=w263:string[])
            n105 = control-ref of="XY Graph"() -> (w268:refnum<vi>)
            n106 = Empty Array?(array=w263) -> (empty?=w274:bool)
            n107 = call "PCB Coverage graph.vi"("UpdatedData"=w261, "error in (no error)"=w250, "XY Graph"=w268, "index"=0, "Disable Autoscale"=w258, "Initialise graph"=TRUE) -> ("error out"=w281:errorcluster)  [unwired: 13 in]
            n108 = Not(x=w274) -> (.not. x?=w273:bool)
            n109 = Select(t=-1 ("Not Tested Components"), s=w274, f=0 ("Not Tested Components")) -> (s? t:f=w271:i32)
            n110 = property on="Not Tested Components" class="LstBox (strict)"(error in=w281, "Item Names"=w263, "Value"=w271, "Top Row"=w279, "Key Focus"=w273) -> (error out=w280:errorcluster)  [unwired: 1 in, 1 out]
            n111 = Select(t=-1 ("Not Tested Components"), s=w273, f=0 ("Not Tested Components")) -> (s? t:f=w270:i32)
            n112 = property on="Not Fitted Components" class="LstBox (strict)"(error in=w280, "Item Names"=w259, "Value"=w270, "Top Row"=w279, "Key Focus"=w274) -> (error out=w283:errorcluster)  [unwired: 1 in, 1 out]
            n113 = property class="Pnl"(reference=w282, error in=w283, "DeferPanUpdts"=FALSE ("Defer Panel Updates")) -> (error out=w284:errorcluster)  [unwired: 1 out]
          }
          event "XY Graph": Mouse Up {
            n114 = event-data() -> ("Coords"=w338:T21, "CtlRef"=w294:refnum<vi>)  [unwired: 1 in]
            n115 = Unbundle By Name(w293) -> ("Not tested components"=w297:string[], "Not fitted components"=w300:string[], "Not Fitted position[x][y]"=w298:dbl[][], "Not Tested position[x][y]"=w299:dbl[][])
            n116 = invoke class="XYGraph (strict)" method="Map Coords To XY"(reference=w294, error in=w291, "Coords"=w338) -> (reference out=w302:refnum<vi>, error out=w301:errorcluster, "XY"=w296:cluster{"X":dbl, "Y":dbl})  [unwired: 4 in, 4 out]
            n117 = property on="Property Node" class="XYGraph (strict)"(reference=w302, error in=w301, "Cursor.Cursor Position"=w296) -> (reference out=w308:refnum<vi>, error out=w309:errorcluster, "Cursor.Cursor Position"=w303:T18, "XScale.Offset"=w335:dbl, "YScale.Offset"=w334:dbl, "XScale.Multiplier"=w333:dbl, "YScale.Multiplier"=w332:dbl)
            n118 = Build Array (concatenate)(w299, w298) -> (w321:dbl[][])
            n119 = Array Size(array=w299) -> (size(s)=w323:i32[])
            n120 = Build Array (concatenate)(w297, w300) -> (w316:string[])
            n121 = Index Array(array=w323) -> (element=w320:i32)  [unwired: 1 in]
            n122 = Index Array(array=w321, index (col) #1=0 ("disabled index (col)")) -> (element #1=w325:dbl[], element #2=w324:dbl[])  [unwired: 3 in]
            n123 = for {
              tunnel: w324 -> [w377] mode=indexing
              tunnel: w325 -> [w378] mode=indexing
              tunnel: [w376] -> w327 mode=indexing
              n124 = Bundle("String"=w378, "String"=w377) -> (w376:cluster{"String":dbl, "String":dbl})  [unwired: 1 in]
            }
            n125 = Bundle("XScale.Offset"=w335, "YScale.Offset"=w334) -> (w330:T22)  [unwired: 1 in]
            n126 = Bundle("XScale.Multiplier"=w333, "YScale.Multiplier"=w332) -> (w295:T23)  [unwired: 1 in]
            n127 = Subtract(x=w303, y=w330) -> (x-y=w331:T18)
            n128 = Divide(x=w331, y=w295) -> (x/y=w319:T18)
            n129 = property on="Property Node" class="XYGraph (strict)"(reference=w308, error in=w309) -> (reference out=w305:refnum<vi>, error out=w307:errorcluster, "AnntList"=w306:T24)
            n130 = Subtract(x=w327, y=w319) -> (x-y=w328:T18[])
            n131 = Re/Im To Polar(2:w319, 3:w328) -> (1:w329:T18[])  [unwired: 1 out]
            n132 = Array Max & Min(array=w329) -> (min index (indices)=w315:i32)  [unwired: 3 out]
            n133 = Index Array(array=w316, index=w315) -> (element=w314:string)
            n134 = Greater?(x=w320, y=w315) -> (0:w322:bool)
            n135 = Unbundle(w319) -> ("Cursor X"=w317:dbl, "Cursor Y"=w318:dbl)
            n136 = Format Into String(format string="%s  (%.3fmm,%.3fmm)", w314, w317, w318) -> (resulting string=w312:string)  [unwired: 2 in, 1 out]
            n137 = case shown="False" w322 {
              tunnel: w307 -> [w353 w366]
              tunnel: w315 -> [w357 w369]
              tunnel: [w363 w368] -> w310
              tunnel: w320 -> [w355 _]
              frame False {
                n138 = Subtract(x=w357, y=w355) -> (x-y=w356:i32)
                n139 = property on="Not Tested\nComponents" class="LstBox (strict)"(error in=w353, "Value"=-1 ("Not Tested Components")) -> (error out=w352:errorcluster)  [unwired: 1 in, 1 out]
                n140 = property on="Not Fitted\n Components" class="LstBox (strict)"(error in=w352) -> (error out=w364:errorcluster, "Number of Rows"=w359:u32, "Top Row"=w358:i32)  [unwired: 1 in, 1 out]
                n141 = Add(x=w359, y=w358) -> (x+y=w361:u32)
                n142 = In Range and Coerce(upper limit=w361, x=w356, lower limit=w358) -> (In Range?=w362:bool)  [unwired: 1 out]
                n143 = Select(t=w358, s=w362, f=w356) -> (s? t:f=w360:i32)
                n144 = property on="Not Fitted \nComponents" class="LstBox (strict)"(error in=w364, "Value"=w356, "Top Row"=w360) -> (error out=w363:errorcluster)  [unwired: 1 in, 1 out]
              }
              frame True {
                n145 = property on="Not Fitted\nComponents" class="LstBox (strict)"(error in=w366, "Value"=-1 ("Not Tested Components")) -> (error out=w365:errorcluster)  [unwired: 1 in, 1 out]
                n146 = property on="Not Tested\nComponents" class="LstBox (strict)"(error in=w365) -> (error out=w375:errorcluster, "Number of Rows"=w372:u32, "Top Row"=w371:i32)  [unwired: 1 in, 1 out]
                n147 = Add(x=w372, y=w371) -> (x+y=w373:u32)
                n148 = In Range and Coerce(upper limit=w373, x=w369, lower limit=w371) -> (In Range?=w374:bool)  [unwired: 1 out]
                n149 = Select(t=w371, s=w374, f=w369) -> (s? t:f=w370:i32)
                n150 = property on="Not Tested\n Components" class="LstBox (strict)"(error in=w375, "Value"=w369, "Top Row"=w370) -> (error out=w368:errorcluster)  [unwired: 1 in, 1 out]
              }
            }
            n151 = in-place {
              in-place-border: w338 -> [w345]
              in-place-border: w312 -> [w344]
              in-place-border: w303 -> [w341]
              in-place-border: w315 -> [w340]
              n152 = in-place-array #1(w306, 0) -> (w346:T25)
              n153 = Bundle By Name(cluster=w346, "Name"=w344, "Index"=w340, "Position"=w345) -> (w343:T25)
              n154 = disable-structure shown="Enabled" {
                disable-tunnel: w343 -> [w350 w351]
                disable-tunnel: [w349 w351] -> w342
                disable-tunnel: w341 -> [w347 _]
                frame Disabled {
                  n155 = call "Fid graph annotation label offset.vi"("Annotation List"=w350, "Load Graph Centre x, y"=FALSE, "Cursor Position"=w347) -> ("Annotation List"=w349:T25)  [unwired: 12 in]
                }
                frame Enabled {
                }
              }
              n156 = in-place-array #1(w342) -> (w304:T24)  [unwired: 1 out]
            }
            n157 = property on="Property Node" class="XYGraph (strict)"(reference=w305, error in=w310, "AnntList"=w304) -> (error out=w292:errorcluster)  [unwired: 1 out]
          }
          event "Save  to file": Value Change {
            n158 = event-data() -> ()  [unwired: 1 in, 1 out]
            n159 = call "File Dialog"("start path"=path "c:/a3di", "default name"="coverage.txt", "error in"=w398, "pattern (all files)"="*.txt") -> ("selected path"=w391:path, "exists"=w392:bool, "cancelled"=w395:bool, "error out"=w394:errorcluster)  [unwired: 8 in]
            n160 = Unbundle By Name(w389) -> ("Control File Relative Path"=w387:path, "Program Name"=w388:string)
            n161 = Unbundle By Name(w383) -> ("Not Fitted position[x][y]"=w381:dbl[][], "Not Tested position[x][y]"=w379:dbl[][], "Not tested components"=w382:string[], "Not fitted components"=w380:string[])
            n162 = case shown="False" w395 {
              tunnel: w394 -> [w407 w426]
              tunnel: [w406 w426] -> w393
              tunnel: w392 -> [w409 _]
              tunnel: w391 -> [w405 _]
              tunnel: w382 -> [w404 _]
              tunnel: w380 -> [w403 _]
              tunnel: w388 -> [w402 _]
              tunnel: w387 -> [w401 _]
              tunnel: w379 -> [w400 _]
              tunnel: w381 -> [w399 _]
              frame False {
                n163 = case shown="True" w409 {
                  tunnel: [TRUE ("T button?") w422] -> w408
                  frame False {
                  }
                  frame True {
                    n164 = Two Button Dialog(message="Do you widh to overwrite file?", 1:"No" ("F button name (\"Cancel\")"), 2:"Yes" ("T button name (\"OK\")")) -> (T button?=w422:bool)
                  }
                }
                n165 = case shown="True" w408 {
                  tunnel: w407 -> [w410 w420]
                  tunnel: [w410 w419] -> w406
                  tunnel: w405 -> [_ w418]
                  tunnel: w404 -> [_ w416]
                  tunnel: w403 -> [_ w415]
                  tunnel: w402 -> [_ w414]
                  tunnel: w401 -> [_ w413]
                  tunnel: w400 -> [_ w412]
                  tunnel: w399 -> [_ w411]
                  frame False {
                  }
                  frame True {
                    n166 = call "Format coverage report.vi"("Not tested components"=w416, "Not Tested position[x][y]"=w412, "Not Fitted position[x][y]"=w411, "TCF File path"=w413, "Not fitted components"=w415, "Program Name"=w414) -> ("Coverage text"=w417:string)  [unwired: 9 in]
                    n167 = Write to Text File(file (use dialog)=w418, text=w417, error in=w420) -> (error out=w419:errorcluster)  [unwired: 1 in, 2 out]
                  }
                }
              }
              frame True {
              }
            }
          }
        }
      }
      frame "Exit" {
        n168 = invoke class="VI" method="FP.Close"(reference=w432, error in=w433) -> (error out=w427:errorcluster)  [unwired: 1 in, 2 out]
      }
    }
  }
  "error out" <- w1
  "Dongle fitted" <- w4
  "XY Graph" <- cluster{dbl[], dbl[]}[] [] ("XY Graph")
